vi "Common Compose Setpoints.vi"(9 "Selected Correctors":u32[](array[numeric]), 11 "Corrector Kicks Subset":dbl[](array[numeric])) -> (3 "Corrector Kicks":dbl[](array[numeric]))   [LabVIEW 2011, in "Common VIs.lvlib"]
doc: "Selects from the complete corrector kick vector (variation vector) the corrector kicks which are being used to FOFB. The unused correctors receives 0."
uses:
  Common VIs.lvlib
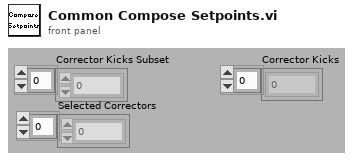
[diagram p1: front panel]
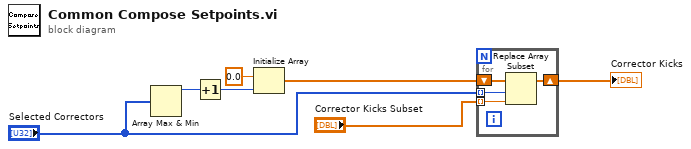
[diagram p0: block diagram]
diagram:
  n1 = Array Max & Min(array="Selected Correctors") -> (max value=w2:u32)  [unwired: 3 out]
  n2 = Increment(x=w2) -> (x+1=w1:u32)
  n3 = Initialize Array(0.0, w1) -> (w6:dbl[])
  n4 = for {
    tunnel: "Corrector Kicks Subset" -> [w8] mode=indexing
    tunnel: "Selected Correctors" -> [w10] mode=indexing
    shift-right: [w9] -> w4
    shift-left: w6 -> [w11]
    n5 = Replace Array Subset(array=w11, new element=w8, index=w10) -> (w9:dbl[])
  }
  "Corrector Kicks" <- w4
